vi "LVClass_HasoSlopes Get Pupil pointeur.vi"(0 "HasoSlopes in":refnum<class "HasoSlopes.lvclass">, 11 "error in (no error)":errorcluster) -> (4 "HasoSlopes out":refnum<class "HasoSlopes.lvclass">, 6 "Pupil id":refnum<class "Pupil.lvclass">, 15 "error out":errorcluster)   [LabVIEW 2020, in "HasoSlopes.lvclass"]
doc: "HasoSlopes pointer to pupil object getter.\n\n--------------------------------------------------------------------------------\n\n<B>HasoSlopesIn </B> : HasoSlopes object.\n<B>HasoSlopesOut </B> : HasoSlopes object.\n<B>Pupil </B> : Pointer to pupil object.\n<B>ErrorIn </B> : Error\n<B>ErrorOut </B> : Error\n\n--------------------------------------------------------------------------------"
uses:
  HasoSlopes.lvclass
  Pupil.lvclass
  HasoSlopes.lvclass/HasoSlopes.ctl
  LVClass_Pupil Write Pupil.vi
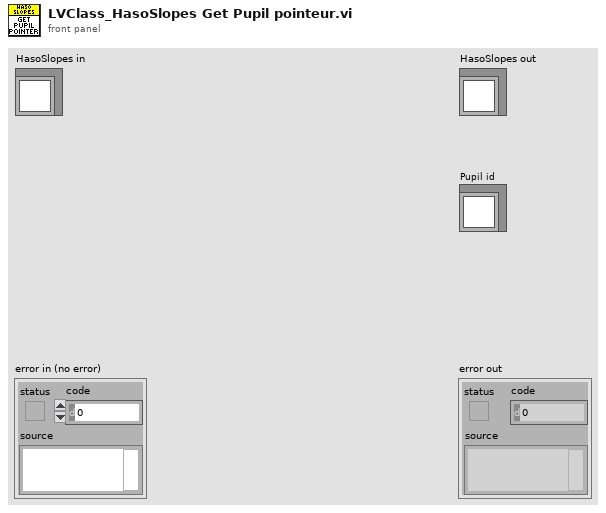
[diagram p1: front panel]
types:
  T1 = typedef "Point2D.ctl" = cluster{"X":u32, "Y":u32}
  T2 = typedef "Point2Df.ctl" = cluster{"X":sgl, "Y":sgl}
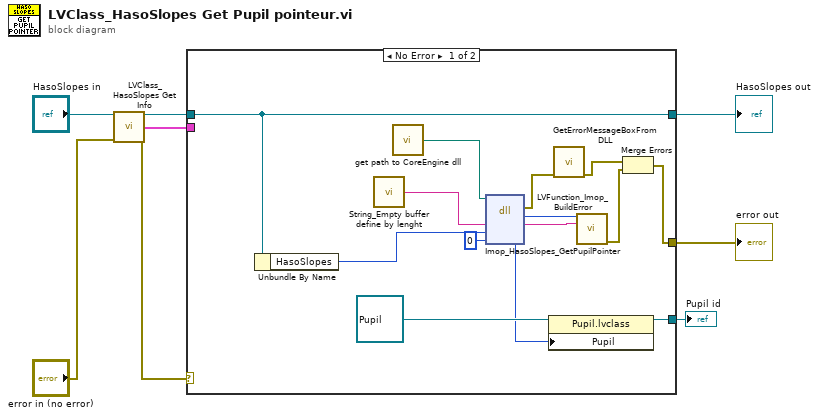
[diagram p0: block diagram]
diagram:
  n1 = call "LVClass_HasoSlopes Get Info.vi"("HasoSlopes in"="HasoSlopes in", "error in (no error)"="error in (no error)") -> ("HasoSlopes out"=w3:refnum<class "HasoSlopes.lvclass">, "dimension"=w2:cluster{"size":T1, "step":T2}, "error out"=w5:errorcluster)  [unwired: 9 in, 2 out]
  n2 = case shown="No Error" w5 {
    selector: w5 -> [_ w24]
    tunnel: [w9 w24] -> w8
    tunnel: [w16 w23] -> w7
    tunnel: w3 -> [w16 w23]
    tunnel: w2 -> [_ _]
    tunnel: [w12 _] -> w1
    frame No Error {
      n3 = Unbundle By Name(w16) -> ("HasoSlopes"=w17:i32)
      n4 = call "String_Empty buffer define by lenght.vi"() -> ("Empty buffer"=w22:string)  [unwired: 1 in]
      n5 = call "get path to CoreEngine dll.vi"() -> ("path to c_interface_vc100.dll"=w19:path)  [unwired: 12 in, 3 out]
      n6 = dll-call lib="D:/2_trunk/Soft_haso/ImOpCoreEngine4_LV2011/DLLs/ImopEngine4_vc100.dll" fn="Imop_HasoSlopes_GetPupilPointer"(path in=w19, "message"=w22, "objet"=w17, "Pupil"=0) -> (error out=w18:errorcluster, "return type"=w20:i32, "message"=w21:string, "Pupil"=w14:i32)  [unwired: 3 in, 1 out]
      n7 = property class="Pupil.lvclass"(reference=refnum<class "Pupil.lvclass"> refnum ("Pupil.lvclass"), "Pupil"=w14) -> (reference out=w12:refnum<class "Pupil.lvclass">)  [unwired: 1 in, 1 out]
      n8 = call "GetErrorMessageBoxFromDLL.vi"("error IN"=w18) -> ("error OUT"=w11:errorcluster)  [unwired: 10 in]
      n9 = call "LVFunction_Imop_BuildError.vi"("code"=w20, "String to Prepend to source (\"\")"=w21) -> ("error out"=w10:errorcluster)  [unwired: 13 in]
      n10 = Merge Errors(w11, w10) -> (w9:errorcluster)
    }
    frame Error {
    }
  }
  "error out" <- w8
  "HasoSlopes out" <- w7
  "Pupil id" <- w1
